vi "Get Default Configuration Parameters.vi"() -> (0 "Default Config Params":variant)   [LabVIEW 2023, in "BLS Cycler Template.lvlib" / "BLS Cycler Template.lvclass"]
uses:
  BLS Cycler Template.lvclass
  Configuration Params.ctl
  <vilib>/ADAS Replay HIL/Template Node/Plugin/Template Node/Common Configuration Params.ctl
  BLS Cycler Template.lvclass/BLS Cycler Template.ctl
  <vilib>/ADAS Replay HIL/Template Node/Plugin/Template Node/Template Node.lvclass
panel:
  # "Set default parameters on the block diagram."
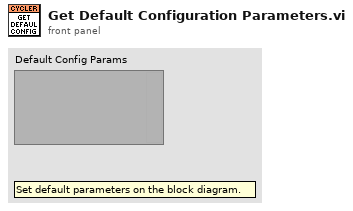
[diagram p1: front panel]
types:
  T1 = typedef "BLS Cycler Template.lvlib/BLS Cycler Template.lvclass/Configuration Params.ctl" = cluster{"Common":T2}
  T2 = typedef "Template Node.lvlib/Template Node.lvclass/Common Configuration Params.ctl" = cluster{"Iteration Interval (s)":dbl, "T0 (ns)":u64, "Priority":i32, "Processor":i32, "Wait in Ready State":bool}
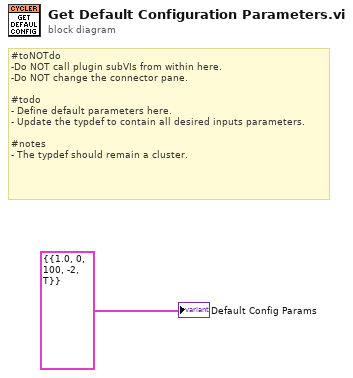
[diagram p0: block diagram]
diagram:
  # "#toNOTdo\n-Do NOT call plugin subVIs from within here.\n-Do NOT change the connector pane.\n\n#todo\n- Define default parameters here.\n- Update the typdef to contain all desired inputs parameters.\n\n#notes\n- The typdef should remain a cluster."
  "Default Config Params" <- T1 {"Common"={"Iteration Interval (s)"=1.0, "T0 (ns)"=0, "Priority"=100, "Processor"=-2, "Wait in Ready State"=TRUE}} ("Default Parameters")
